vi "get outgoing object Information element by name.vi"(10 "name":string, 11 "object info":T1) -> (1 "found":bool, 3 "element out":dbl)   [LabVIEW 2019, in "HLA Custom Device Engine.lvlib"]
uses:
  HLA Custom Device Engine.lvlib
  _typedefs/object_info_outgoing_type.ctl
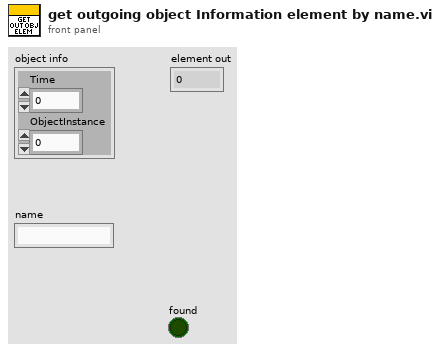
[diagram p1: front panel]
types:
  T1 = typedef "HLA Custom Device Engine.lvlib/object_info_outgoing_type.ctl" = cluster{"Time":dbl, "ObjectInstance":u64}
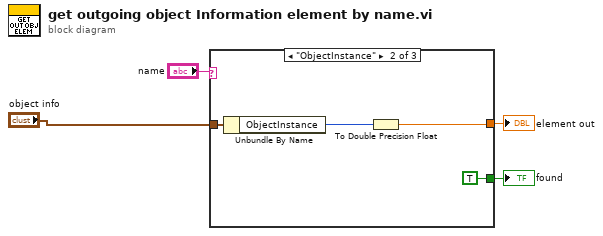
[diagram p0: block diagram]
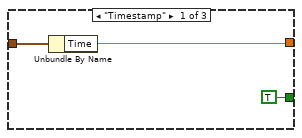
[diagram p2: hidden frame]
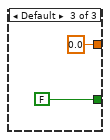
[diagram p3: hidden frame]
diagram:
  n1 = case shown="\"ObjectInstance\"" "name" {
    tunnel: "object info" -> [w6 w10 _]
    tunnel: [w7 w8 0.0] -> w2
    tunnel: [TRUE TRUE FALSE] -> w1
    frame "Timestamp" {
      n2 = Unbundle By Name(w6) -> ("Time"=w7:dbl)
    }
    frame "ObjectInstance" {
      n3 = Unbundle By Name(w10) -> ("ObjectInstance"=w11:u64)
      n4 = To Double Precision Float(number=w11) -> (double precision float=w8:dbl)
    }
    frame Default {
    }
  }
  "element out" <- w2
  "found" <- w1
